vi "Physical Constant Configuration.vi"() -> ()   [LabVIEW 2013]
panel:
  in  "Minimum Z Extension (nm)":dbl
  in  "Maximum Z Extension (nm)":dbl
  in  "Z Piezo Response (nm/V)":dbl
  in  "Minimum Y Extension (nm)":dbl
  in  "Maximum Y Extension (nm)":dbl
  in  "Y Piezo Response (nm/V)":dbl
  in  "Minimum X Extension (nm)":dbl
  in  "Maximum X Extension (nm)":dbl
  in  "X Piezo Response (nm/V)":dbl
  in  "Minimum Output Voltage (V)":dbl
  in  "Maximum Output Voltage (V)":dbl
  in  "Minimum Input Voltage (V)":dbl
  in  "Maximum Input Voltage (V)":dbl
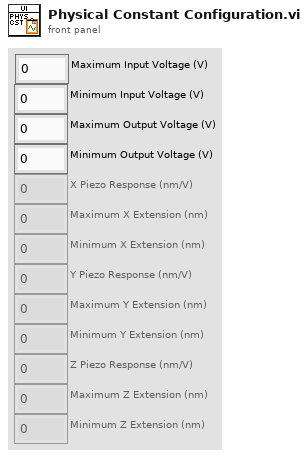
[diagram p1: front panel]
types:
  T1 = enum8{"Enabled", "Disabled", "Disabled and Grayed Out"}
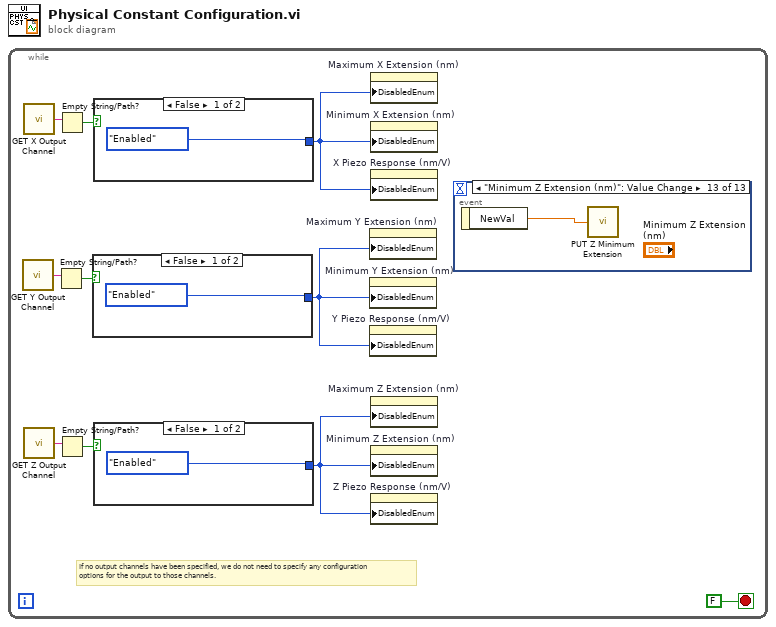
[diagram p0: block diagram]
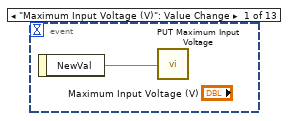
[diagram p2: hidden frame]
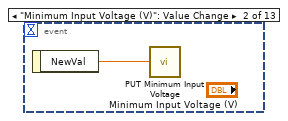
[diagram p3: hidden frame]
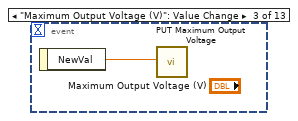
[diagram p4: hidden frame]
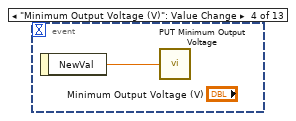
[diagram p5: hidden frame]
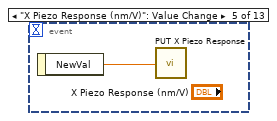
[diagram p6: hidden frame]
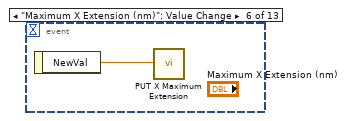
[diagram p7: hidden frame]
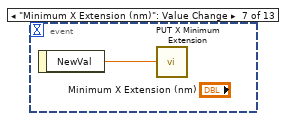
[diagram p8: hidden frame]
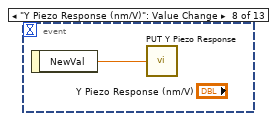
[diagram p9: hidden frame]
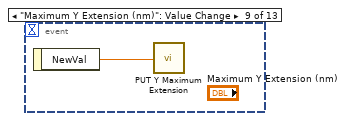
[diagram p10: hidden frame]
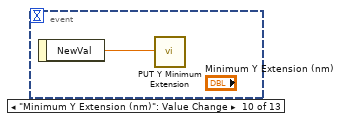
[diagram p11: hidden frame]
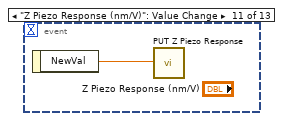
[diagram p12: hidden frame]
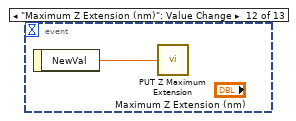
[diagram p13: hidden frame]
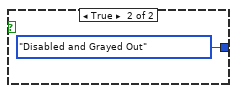
[diagram p14: hidden frame]
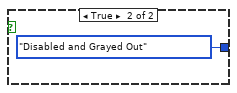
[diagram p15: hidden frame]
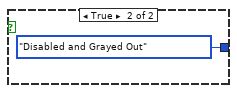
[diagram p16: hidden frame]
diagram:
  n1 = while {
    stop <- FALSE stop-if-true
    # "If no output channels have been specified, we do not need to specify any configuration\noptions for the output to those channels."
    n2 = call "GET Y Output Channel.vi"() -> ("Y Output Channel"=w7:string)
    n3 = call "GET X Output Channel.vi"() -> ("X Output Channel"=w10:string)
    n4 = call "GET Z Output Channel.vi"() -> ("Z Output Channel"=w3:string)
    n5 = Empty String/Path?(string/path=w7) -> (empty?=w6:bool)
    n6 = Empty String/Path?(string/path=w10) -> (empty?=w9:bool)
    n7 = Empty String/Path?(string/path=w3) -> (empty?=w2:bool)
    n8 = case shown="False" w6 {
      tunnel: [T1."Enabled" ("Disabled") T1."Disabled and Grayed Out" ("Disabled")] -> w5
      frame False {
      }
      frame True {
      }
    }
    n9 = case shown="False" w9 {
      tunnel: [T1."Enabled" ("Disabled") T1."Disabled and Grayed Out" ("Disabled")] -> w8
      frame False {
      }
      frame True {
      }
    }
    n10 = case shown="False" w2 {
      tunnel: [T1."Enabled" ("Disabled") T1."Disabled and Grayed Out" ("Disabled")] -> w1
      frame False {
      }
      frame True {
      }
    }
    n11 = property on="Maximum Y Extension (nm)" class="DigNum (strict)"("DisabledEnum"=w5) -> ()  [unwired: 2 in, 2 out]
    n12 = property on="Minimum Y Extension (nm)" class="DigNum (strict)"("DisabledEnum"=w5) -> ()  [unwired: 2 in, 2 out]
    n13 = property on="Y Piezo Response (nm/V)" class="DigNum (strict)"("DisabledEnum"=w5) -> ()  [unwired: 2 in, 2 out]
    n14 = property on="Maximum X Extension (nm)" class="DigNum (strict)"("DisabledEnum"=w8) -> ()  [unwired: 2 in, 2 out]
    n15 = property on="Minimum X Extension (nm)" class="DigNum (strict)"("DisabledEnum"=w8) -> ()  [unwired: 2 in, 2 out]
    n16 = property on="X Piezo Response (nm/V)" class="DigNum (strict)"("DisabledEnum"=w8) -> ()  [unwired: 2 in, 2 out]
    n17 = property on="Maximum Z Extension (nm)" class="DigNum (strict)"("DisabledEnum"=w1) -> ()  [unwired: 2 in, 2 out]
    n18 = property on="Minimum Z Extension (nm)" class="DigNum (strict)"("DisabledEnum"=w1) -> ()  [unwired: 2 in, 2 out]
    n19 = property on="Z Piezo Response (nm/V)" class="DigNum (strict)"("DisabledEnum"=w1) -> ()  [unwired: 2 in, 2 out]
    n20 = event shown="[12] \"Minimum Z Extension (nm)\": Value Change" {
      selector: _ -> [_ _ _ _ _ _ _ _ _ _ _ _ _]
      dyn-events: _ -> [_ _ _ _ _ _ _ _ _ _ _ _ _]
      timeout: _ -> [_ _ _ _ _ _ _ _ _ _ _ _ _]
      event "Maximum Input Voltage (V)": Value Change {
        n21 = event-data() -> ("NewVal"=w11:dbl)  [unwired: 1 in]
        n22 = call "PUT Maximum Input Voltage.vi"("Maximum Input Voltage"=w11) -> ()
      }
      event "Minimum Input Voltage (V)": Value Change {
        n23 = event-data() -> ("NewVal"=w12:dbl)  [unwired: 1 in]
        n24 = call "PUT Minimum Input Voltage.vi"("Minimum Input Voltage"=w12) -> ()
      }
      event "Maximum Output Voltage (V)": Value Change {
        n25 = event-data() -> ("NewVal"=w13:dbl)  [unwired: 1 in]
        n26 = call "PUT Maximum Output Voltage.vi"("Maximum Output Voltage"=w13) -> ()
      }
      event "Minimum Output Voltage (V)": Value Change {
        n27 = event-data() -> ("NewVal"=w14:dbl)  [unwired: 1 in]
        n28 = call "PUT Minimum Output Voltage.vi"("Minimum Output Voltage"=w14) -> ()
      }
      event "X Piezo Response (nm/V)": Value Change {
        n29 = event-data() -> ("NewVal"=w15:dbl)  [unwired: 1 in]
        n30 = call "PUT X Piezo Response.vi"("X Piezo Response"=w15) -> ()
      }
      event "Maximum X Extension (nm)": Value Change {
        n31 = event-data() -> ("NewVal"=w16:dbl)  [unwired: 1 in]
        n32 = call "PUT X Maximum Extension.vi"("X Maximum Extension"=w16) -> ()
      }
      event "Minimum X Extension (nm)": Value Change {
        n33 = event-data() -> ("NewVal"=w17:dbl)  [unwired: 1 in]
        n34 = call "PUT X Minimum Extension.vi"("X Minimum Extension"=w17) -> ()
      }
      event "Y Piezo Response (nm/V)": Value Change {
        n35 = event-data() -> ("NewVal"=w18:dbl)  [unwired: 1 in]
        n36 = call "PUT Y Piezo Response.vi"("Y Piezo Response"=w18) -> ()
      }
      event "Maximum Y Extension (nm)": Value Change {
        n37 = event-data() -> ("NewVal"=w19:dbl)  [unwired: 1 in]
        n38 = call "PUT Y Maximum Extension.vi"("Y Maximum Extension"=w19) -> ()
      }
      event "Minimum Y Extension (nm)": Value Change {
        n39 = event-data() -> ("NewVal"=w20:dbl)  [unwired: 1 in]
        n40 = call "PUT Y Minimum Extension.vi"("Y Minimum Extension"=w20) -> ()
      }
      event "Z Piezo Response (nm/V)": Value Change {
        n41 = event-data() -> ("NewVal"=w21:dbl)  [unwired: 1 in]
        n42 = call "PUT Z Piezo Response.vi"("Z Piezo Response"=w21) -> ()
      }
      event "Maximum Z Extension (nm)": Value Change {
        n43 = event-data() -> ("NewVal"=w22:dbl)  [unwired: 1 in]
        n44 = call "PUT Z Maximum Extension.vi"("Z Maximum Extension"=w22) -> ()
      }
      event "Minimum Z Extension (nm)": Value Change {
        n45 = event-data() -> ("NewVal"=w23:dbl)  [unwired: 1 in]
        n46 = call "PUT Z Minimum Extension.vi"("Z Minimum Extension"=w23) -> ()
      }
    }
  }
